vi "ServiceRegister_Set.vi"(8 "Fehler (Eingang, kein Fehler)":errorcluster caption="Error_In", 10 "Register Value (0..255)":u8, 11 "OXYGEN Ref In":refnum<visa-resource-name>) -> (0 "Fehler (Ausgang)":errorcluster caption="Error_Out", 1 "communication_data":T1, 3 "OXYGEN Ref Out":refnum<visa-resource-name>)   [LabVIEW 2018, in "OXYGEN.lvlib"]
doc: "Sets the service request enable register."
uses:
  OXYGEN.lvlib
  TypeDefs/Cluster_RawCommData.ctl
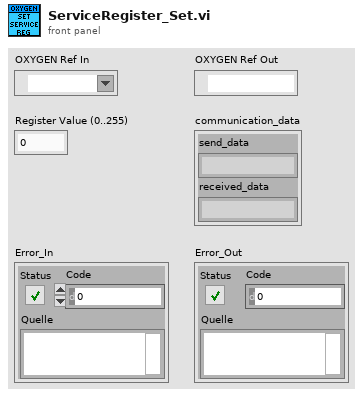
[diagram p1: front panel]
types:
  T1 = typedef "OXYGEN.lvlib/Cluster_RawCommData.ctl" = cluster{"send_data":string, "received_data":string}
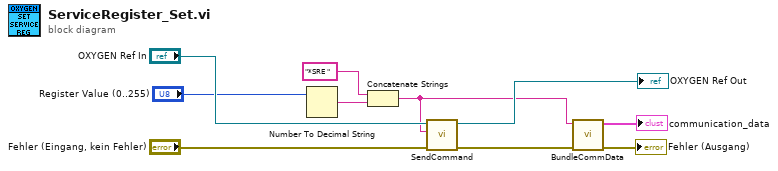
[diagram p0: block diagram]
diagram:
  n1 = Number To Decimal String(number="Register Value (0..255)") -> (decimal integer string=w3:string)  [unwired: 1 in]
  n2 = Concatenate Strings("*SRE " ("Schreibpuffer"), w3) -> (w1:string)
  n3 = call "SendCommand.vi"("error in (no error)"="Fehler (Eingang, kein Fehler)", "String to Send"=w1, "OXY_SCPI Reseource In"="OXYGEN Ref In") -> ("error out"=w6:errorcluster, "OXY_SCPI Reseource Out"=→"OXYGEN Ref Out":refnum<visa-resource-name>)  [unwired: 7 in]
  n4 = call "BundleCommData.vi"("error in (no error)"=w6, "send_data"=w1) -> ("error out"=→"Fehler (Ausgang)":errorcluster, "communication_data"=→"communication_data":T1)  [unwired: 8 in]
